vi "Measure Voltage.vi"(8 "error in (no error)":errorcluster, 11 "Low Level PSU In":refnum<class "Low Level PSU.lvclass">) -> (0 "error out":errorcluster, 2 "Output Voltage":dbl format="%.4f", 3 "Low Level PSU Out":refnum<class "Low Level PSU.lvclass">)   [LabVIEW 2020, in "Low Level PSU.lvlib" / "Low Level PSU.lvclass"]
uses:
  Low Level PSU.lvclass
  Low Level PSU.lvclass/Low Level PSU.ctl
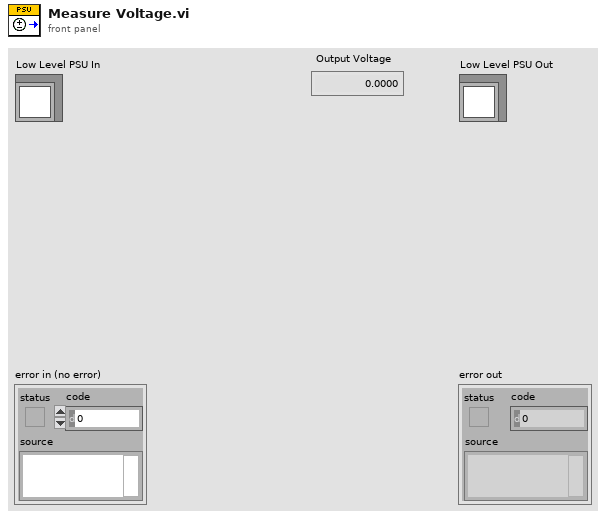
[diagram p1: front panel]
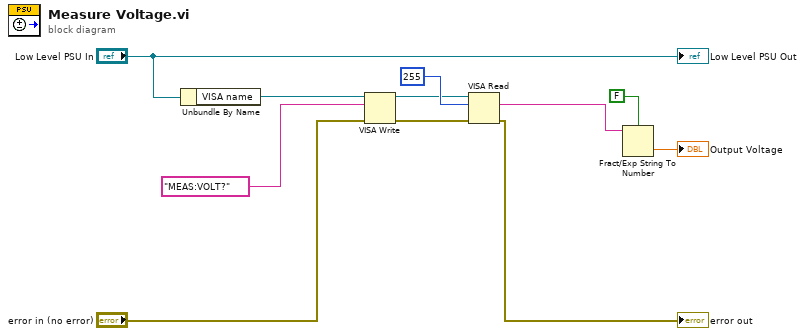
[diagram p0: block diagram]
diagram:
  n1 = Unbundle By Name("Low Level PSU In") -> ("VISA name"=w5:refnum<visa-resource-name>)
  n2 = VISA Write(VISA resource name=w5, write buffer="MEAS:VOLT?" ("format string"), error in (no error)="error in (no error)") -> (VISA resource name out=w10:refnum<visa-resource-name>, error out=w9:errorcluster)  [unwired: 1 out]
  n3 = VISA Read(VISA resource name=w10, byte count=u32 255 ("byte count (0)"), error in (no error)=w9) -> (read buffer=w1:string, error out=→"error out":errorcluster)  [unwired: 2 out]
  n4 = Fract/Exp String To Number(use system decimal point (T)=FALSE, string=w1) -> (number=→"Output Voltage":dbl)  [unwired: 2 in, 1 out]
  "Low Level PSU Out" <- "Low Level PSU In"
